vi "Drive_Utils_RelativeXYtoAbsolute.vi"(4 "error in":errorcluster, 5 "Angle":dbl, 6 "Y":dbl, 7 "X":dbl) -> (0 "error out":errorcluster, 2 "Y":dbl, 3 "X":dbl)   [LabVIEW 2009, in "Drive.lvlib" / "Drive_Utils.lvlib"]
uses:
  Drive_Utils.lvlib
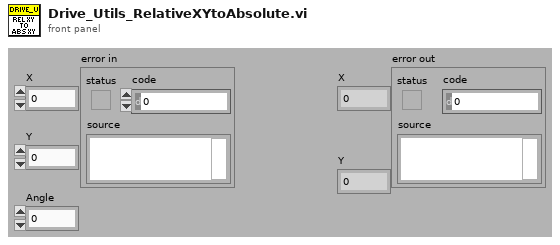
[diagram p1: front panel]
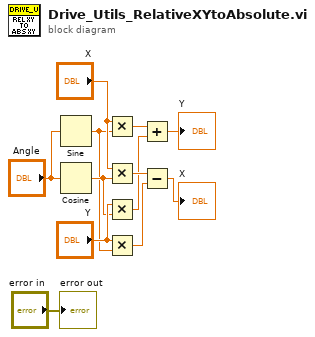
[diagram p0: block diagram]
diagram:
  n1 = Sine(x="Angle") -> (sin(x)=w8:dbl)
  n2 = Cosine(x="Angle") -> (cos(x)=w9:dbl)
  n3 = Multiply(x="X", y=w8) -> (x*y=w4:dbl)
  n4 = Multiply(x="X", y=w9) -> (x*y=w7:dbl)
  n5 = Multiply(x="Y", y=w9) -> (x*y=w3:dbl)
  n6 = Multiply(x="Y", y=w8) -> (x*y=w6:dbl)
  n7 = Add(x=w4, y=w3) -> (x+y=→"Y":dbl)
  n8 = Subtract(x=w7, y=w6) -> (x-y=→"X":dbl)
  "error out" <- "error in"
